vi "Obtain.vi"(8 "Error In":errorcluster, 11 "Object Name":string) -> (0 "Error Out":errorcluster, 2 "Found?":bool, 3 "Object Reference":refnum<class "CS++Reference.lvclass">)   [LabVIEW 2015, in "CS++BaseClasses.lvlib" / "CS++Reference.lvclass"]
doc: "Obtain an object reference from object name."
uses:
  CS++Reference.lvclass
  Base/CS++Base.lvclass
  CS++Reference.lvclass/CS++Reference.ctl
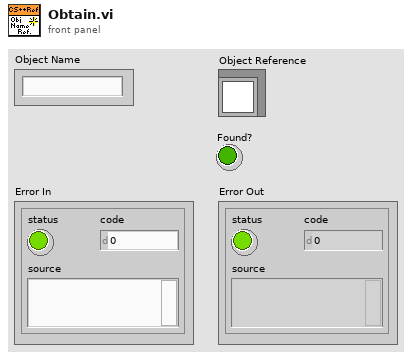
[diagram p1: front panel]
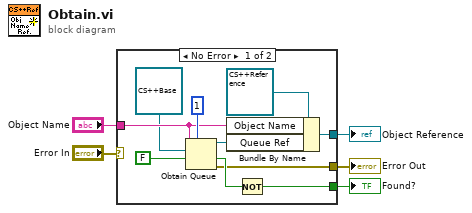
[diagram p0: block diagram]
diagram:
  n1 = case shown="No Error" "Error In" {
    selector: "Error In" -> [_ w16]
    tunnel: "Object Name" -> [w11 _]
    tunnel: [w10 w16] -> w4
    tunnel: [w6 _] -> w3
    tunnel: [w13 _] -> w1
    frame No Error {
      n2 = Obtain Queue(max queue size (-1, unlimited)=1, name (unnamed)=w11, element data type=refnum<class "CS++Base.lvclass"> refnum ("CS++BaseClasses.lvlib:CS++Base.lvclass"), create if not found? (T)=FALSE) -> (queue out=w7:refnum<queue>, created new?=w14:bool, error out=w10:errorcluster)  [unwired: 1 in]
      n3 = Bundle By Name(cluster=refnum<class "CS++Reference.lvclass"> refnum ("CS++BaseClasses.lvlib:CS++Reference.lvclass"), "Object Name"=w11, "Queue Ref"=w7) -> (w13:refnum<class "CS++Reference.lvclass">)
      n4 = Not(x=w14) -> (.not. x?=w6:bool)
    }
    frame Error {
    }
  }
  "Error Out" <- w4
  "Found?" <- w3
  "Object Reference" <- w1
